vi "Get Value (String).vi"(8 "error in (no error)":errorcluster, 10 "Name":string, 11 "Camera in":refnum<class "Camera.lvclass">) -> (0 "error out":errorcluster, 2 "Value":string, 3 "Camera":refnum<class "Camera.lvclass">)   [LabVIEW 2020, in "Camera.lvclass"]
uses:
  Camera.lvclass
  Camera.lvclass/Camera.ctl
  <vilib>/Utility/error.llb/Error Cluster From Error Code.vi
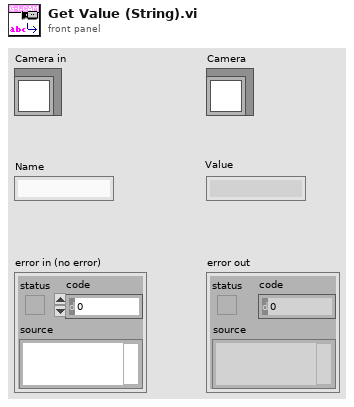
[diagram p1: front panel]
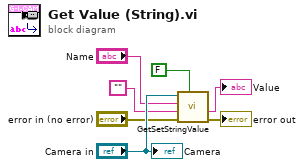
[diagram p0: block diagram]
diagram:
  n1 = call "GetSetStringValue.vi"("Set?"=FALSE, "error in (no error)"="error in (no error)", "Value In"="", "Name"="Name", "Camera in"="Camera in") -> ("error out"=→"error out":errorcluster, "Value Out"=→"Value":string)  [unwired: 5 in]
  "Camera" <- "Camera in"
